vi "MKS MW.vi"() -> ()   [LabVIEW 2015]
doc: "Example VI that demonstrates all library features."
uses:
  PL MKS MW.lvclass
panel:
  in  "port":refnum<visa-resource-name>
  in  "set auto preset":bool
  in  "auto mode preset index":u8(ring) items=["0", "1", "2", "3", "4", "5", "6", "7", "8", "9", "A", "B", "C"]
  in  "recall preset":bool
  in  "store preset":bool
  in  "store/recall preset index":u8(ring) items=["0", "1", "2", "3", "4", "5", "6", "7", "8", "9"]
  in  "decrement preset":bool
  in  "increment preset":bool
  in  "decrement C2":bool
  in  "increment C2":bool
  in  "decrement C1":bool
  in  "increment C1":bool
  out "power on time":u32 format="%<%H:%M:%S>t"
  out "faults":T1
  out "software version":string
  out "preset index":u8(ring) items=["0", "1", "2", "3", "4", "5", "6", "7", "8", "9", "A", "B", "C"]
  in  "control mode":u16(ring)=1 items=["manual"=1, "analog"=2, "auto"=3]
  in  "C2, %":u8
  in  "C1, %":u8
  out "Upp, V":u16
  out "Udc, V":u16
  out "MKS":refnum<class "PL MKS MW.lvclass">
  in  "stop bits":u16(ring)=10 items=["1.0"=10, "1.5"=15, "2.0"=20]
  in  "parity":u16(ring) items=["None", "Odd", "Even", "Mark", "Space"]
  in  "data bits":u16=8
  in  "baud rate":u32=9600
  out "error":errorcluster
  in  "stop":bool
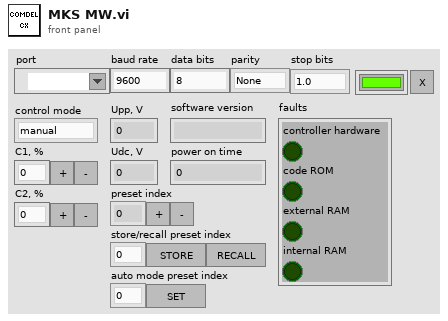
[diagram p1: front panel]
types:
  T1 = cluster{"controller hardware":bool, "code ROM":bool, "external RAM":bool, "internal RAM":bool}
  T2 = cluster{"Udc, V":u16, "Upp, V":u16, "C1, %":u8, "C2, %":u8, "control mode":u16, "preset index":u8}
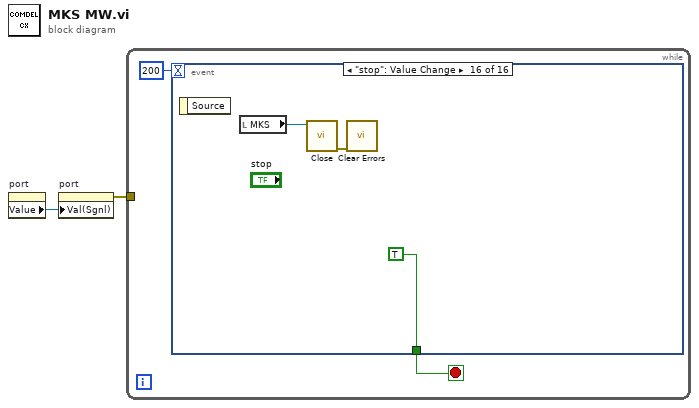
[diagram p0: block diagram]
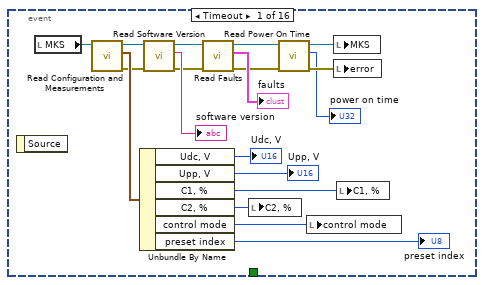
[diagram p2: hidden frame]
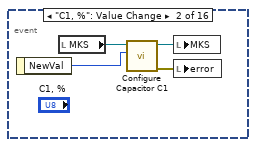
[diagram p3: hidden frame]
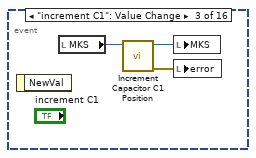
[diagram p4: hidden frame]
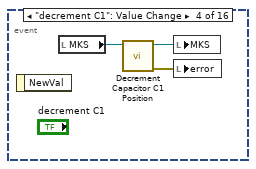
[diagram p5: hidden frame]
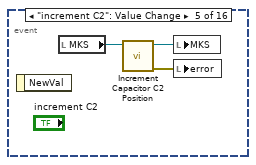
[diagram p6: hidden frame]
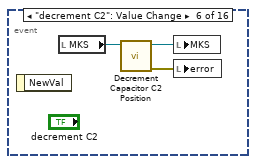
[diagram p7: hidden frame]
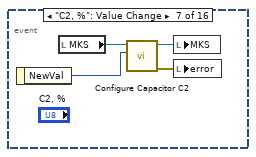
[diagram p8: hidden frame]
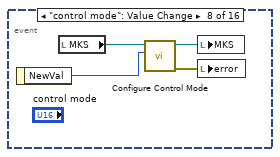
[diagram p9: hidden frame]
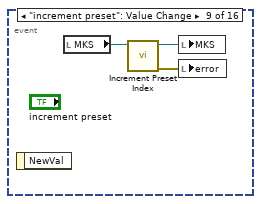
[diagram p10: hidden frame]
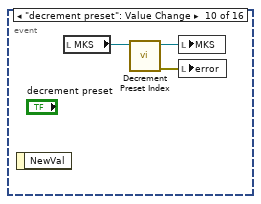
[diagram p11: hidden frame]
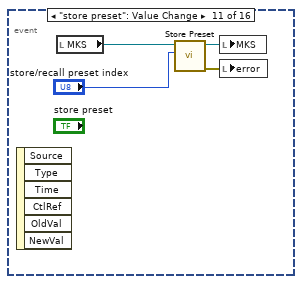
[diagram p12: hidden frame]
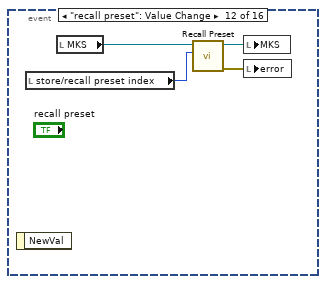
[diagram p13: hidden frame]
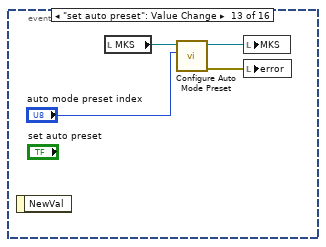
[diagram p14: hidden frame]
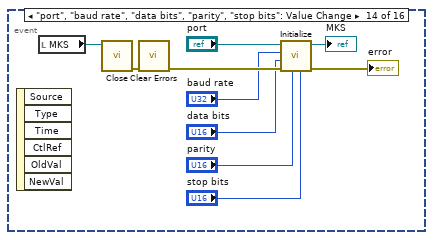
[diagram p15: hidden frame]
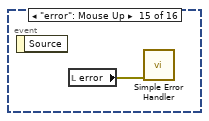
[diagram p16: hidden frame]
diagram:
  n1 = property on="port" class="VISAName"() -> ("Value"=w1:refnum<visa-resource-name>)  [unwired: 2 in, 2 out]
  n2 = property on="port" class="VISAName"("Val(Sgnl)"=w1) -> (error out=w2:errorcluster)  [unwired: 2 in, 1 out]
  n3 = while {
    tunnel: w2 -> [_]
    stop <- w3 stop-if-true
    n4 = event shown="[15] \"stop\": Value Change" {
      selector: _ -> [_ _ _ _ _ _ _ _ _ _ _ _ _ _ _ _]
      dyn-events: _ -> [_ _ _ _ _ _ _ _ _ _ _ _ _ _ _ _]
      timeout: 200 -> [_ _ _ _ _ _ _ _ _ _ _ _ _ _ _ _]
      tunnel: [_ _ _ _ _ _ _ _ _ _ _ _ _ _ _ TRUE ("stop")] -> w3
      event Timeout {
        n5 = event-data() -> ()  [unwired: 1 in, 1 out]
        n6 = local read "MKS"() -> (w23:refnum<class "PL MKS MW.lvclass">)
        n7 = call "Read Configuration and Measurements.vi"("MKS MW in"=w23) -> ("error out"=w17:errorcluster, "configuration and measurements"=w21:T2, "MKS MW out"=w22:refnum<class "PL MKS MW.lvclass">)  [unwired: 8 in]
        n8 = Unbundle By Name(w21) -> ("Udc, V"=→"Udc, V":u16, "Upp, V"=→"Upp, V":u16, "C1, %"=w20:u8, "C2, %"=w19:u8, "control mode"=w18:u16, "preset index"=→"preset index":u8)
        n9 = call "Read Software Version.vi"("error in (no error)"=w17, "MKS MW in"=w22) -> ("error out"=w14:errorcluster, "software version"=→"software version":string, "MKS MW out"=w16:refnum<class "PL MKS MW.lvclass">)  [unwired: 7 in]
        n10 = call "Read Faults.vi"("error in (no error)"=w14, "MKS MW in"=w16) -> ("error out"=w11:errorcluster, "faults"=→"faults":T1, "MKS MW out"=w12:refnum<class "PL MKS MW.lvclass">)  [unwired: 7 in]
        n11 = local write "C2, %"(w19) -> ()
        n12 = call "Read Power On Time.vi"("error in (no error)"=w11, "MKS MW in"=w12) -> ("error out"=w10:errorcluster, "power on time, s"=→"power on time":u32, "MKS MW out"=w9:refnum<class "PL MKS MW.lvclass">)  [unwired: 7 in]
        n13 = local write "control mode"(w18) -> ()
        n14 = local write "MKS"(w9) -> ()
        n15 = local write "error"(w10) -> ()
        n16 = local write "C1, %"(w20) -> ()
      }
      event "C1, %": Value Change {
        n17 = event-data() -> ("NewVal"=w24:u8)  [unwired: 1 in]
        n18 = local read "MKS"() -> (w25:refnum<class "PL MKS MW.lvclass">)
        n19 = call "Configure Capacitor C1.vi"("position, %"=w24, "MKS MW in"=w25) -> ("error out"=w27:errorcluster, "MKS MW out"=w26:refnum<class "PL MKS MW.lvclass">)  [unwired: 8 in]
        n20 = local write "MKS"(w26) -> ()
        n21 = local write "error"(w27) -> ()
      }
      event "increment C1": Value Change {
        n22 = event-data() -> ()  [unwired: 1 in, 1 out]
        n23 = local read "MKS"() -> (w29:refnum<class "PL MKS MW.lvclass">)
        n24 = call "Increment Capacitor C1 Position.vi"("MKS MW in"=w29) -> ("error out"=w30:errorcluster, "MKS MW out"=w28:refnum<class "PL MKS MW.lvclass">)  [unwired: 9 in]
        n25 = local write "MKS"(w28) -> ()
        n26 = local write "error"(w30) -> ()
      }
      event "decrement C1": Value Change {
        n27 = event-data() -> ()  [unwired: 1 in, 1 out]
        n28 = local read "MKS"() -> (w31:refnum<class "PL MKS MW.lvclass">)
        n29 = call "Decrement Capacitor C1 Position.vi"("MKS MW in"=w31) -> ("error out"=w33:errorcluster, "MKS MW out"=w32:refnum<class "PL MKS MW.lvclass">)  [unwired: 9 in]
        n30 = local write "MKS"(w32) -> ()
        n31 = local write "error"(w33) -> ()
      }
      event "increment C2": Value Change {
        n32 = event-data() -> ()  [unwired: 1 in, 1 out]
        n33 = local read "MKS"() -> (w34:refnum<class "PL MKS MW.lvclass">)
        n34 = call "Increment Capacitor C2 Position.vi"("MKS MW in"=w34) -> ("error out"=w36:errorcluster, "MKS MW out"=w35:refnum<class "PL MKS MW.lvclass">)  [unwired: 9 in]
        n35 = local write "MKS"(w35) -> ()
        n36 = local write "error"(w36) -> ()
      }
      event "decrement C2": Value Change {
        n37 = event-data() -> ()  [unwired: 1 in, 1 out]
        n38 = local read "MKS"() -> (w37:refnum<class "PL MKS MW.lvclass">)
        n39 = call "Decrement Capacitor C2 Position.vi"("MKS MW in"=w37) -> ("error out"=w39:errorcluster, "MKS MW out"=w38:refnum<class "PL MKS MW.lvclass">)  [unwired: 9 in]
        n40 = local write "MKS"(w38) -> ()
        n41 = local write "error"(w39) -> ()
      }
      event "C2, %": Value Change {
        n42 = event-data() -> ("NewVal"=w40:u8)  [unwired: 1 in]
        n43 = local read "MKS"() -> (w41:refnum<class "PL MKS MW.lvclass">)
        n44 = call "Configure Capacitor C2.vi"("position, %"=w40, "MKS MW in"=w41) -> ("error out"=w43:errorcluster, "MKS MW out"=w42:refnum<class "PL MKS MW.lvclass">)  [unwired: 8 in]
        n45 = local write "MKS"(w42) -> ()
        n46 = local write "error"(w43) -> ()
      }
      event "control mode": Value Change {
        n47 = event-data() -> ("NewVal"=w44:u16)  [unwired: 1 in]
        n48 = local read "MKS"() -> (w45:refnum<class "PL MKS MW.lvclass">)
        n49 = call "Configure Control Mode.vi"("control mode"=w44, "MKS MW in"=w45) -> ("error out"=w46:errorcluster, "MKS MW out"=w47:refnum<class "PL MKS MW.lvclass">)  [unwired: 8 in]
        n50 = local write "MKS"(w47) -> ()
        n51 = local write "error"(w46) -> ()
      }
      event "increment preset": Value Change {
        n52 = event-data() -> ()  [unwired: 1 in, 1 out]
        n53 = local read "MKS"() -> (w48:refnum<class "PL MKS MW.lvclass">)
        n54 = call "Increment Preset Index.vi"("MKS MW in"=w48) -> ("error out"=w50:errorcluster, "MKS MW out"=w49:refnum<class "PL MKS MW.lvclass">)  [unwired: 9 in]
        n55 = local write "MKS"(w49) -> ()
        n56 = local write "error"(w50) -> ()
      }
      event "decrement preset": Value Change {
        n57 = event-data() -> ()  [unwired: 1 in, 1 out]
        n58 = local read "MKS"() -> (w51:refnum<class "PL MKS MW.lvclass">)
        n59 = call "Decrement Preset Index.vi"("MKS MW in"=w51) -> ("error out"=w53:errorcluster, "MKS MW out"=w52:refnum<class "PL MKS MW.lvclass">)  [unwired: 9 in]
        n60 = local write "MKS"(w52) -> ()
        n61 = local write "error"(w53) -> ()
      }
      event "store preset": Value Change {
        n62 = event-data() -> ()  [unwired: 1 in, 6 out]
        n63 = local read "MKS"() -> (w57:refnum<class "PL MKS MW.lvclass">)
        n64 = call "Store Preset.vi"("preset index"="store/recall preset index", "MKS MW in"=w57) -> ("error out"=w55:errorcluster, "MKS MW out"=w56:refnum<class "PL MKS MW.lvclass">)  [unwired: 8 in]
        n65 = local write "MKS"(w56) -> ()
        n66 = local write "error"(w55) -> ()
      }
      event "recall preset": Value Change {
        n67 = event-data() -> ()  [unwired: 1 in, 1 out]
        n68 = local read "store/recall preset index"() -> (w58:u8)
        n69 = local read "MKS"() -> (w61:refnum<class "PL MKS MW.lvclass">)
        n70 = call "Recall Preset.vi"("preset index"=w58, "MKS MW in"=w61) -> ("error out"=w59:errorcluster, "MKS MW out"=w60:refnum<class "PL MKS MW.lvclass">)  [unwired: 8 in]
        n71 = local write "MKS"(w60) -> ()
        n72 = local write "error"(w59) -> ()
      }
      event "set auto preset": Value Change {
        n73 = event-data() -> ()  [unwired: 1 in, 1 out]
        n74 = local read "MKS"() -> (w65:refnum<class "PL MKS MW.lvclass">)
        n75 = call "Configure Auto Mode Preset.vi"("preset index"="auto mode preset index", "MKS MW in"=w65) -> ("error out"=w63:errorcluster, "MKS MW out"=w64:refnum<class "PL MKS MW.lvclass">)  [unwired: 8 in]
        n76 = local write "MKS"(w64) -> ()
        n77 = local write "error"(w63) -> ()
      }
      event "port", "baud rate", "data bits", "parity", "stop bits": Value Change {
        n78 = event-data() -> ()  [unwired: 1 in, 6 out]
        n79 = local read "MKS"() -> (w75:refnum<class "PL MKS MW.lvclass">)
        n80 = call "Close.vi"("MKS MW in"=w75) -> ("error out"=w68:errorcluster)  [unwired: 10 in]
        n81 = call <vilib>:"Clear Errors.vi"("error in (no error)"=w68) -> ("error out"=w73:errorcluster)  [unwired: 5 in, 1 out]
        n82 = call "Initialize.vi"("stop bits (1.0)"="stop bits", "parity (none)"="parity", "error in (no error)"=w73, "data bits (8)"="data bits", "baud rate (9600)"="baud rate", "port"="port") -> ("error out"=→"error":errorcluster, "MKS MW out"=→"MKS":refnum<class "PL MKS MW.lvclass">)  [unwired: 4 in]
      }
      event "error": Mouse Up {
        n83 = event-data() -> ()  [unwired: 1 in, 1 out]
        n84 = local read "error"() -> (w76:errorcluster)
        n85 = call <vilib>:"Simple Error Handler.vi"("error in (no error)"=w76) -> ()  [unwired: 4 in, 5 out]
      }
      event "stop": Value Change {
        n86 = event-data() -> ()  [unwired: 1 in, 1 out]
        n87 = local read "MKS"() -> (w78:refnum<class "PL MKS MW.lvclass">)
        n88 = call "Close.vi"("MKS MW in"=w78) -> ("error out"=w77:errorcluster)  [unwired: 10 in]
        n89 = call <vilib>:"Clear Errors.vi"("error in (no error)"=w77) -> ()  [unwired: 5 in, 2 out]
      }
    }
  }
